vi "DefaultPsTactic.vi"(9 "Game in":refnum<class "Game.lvclass">, 10 "Robot":refnum<class "Robot.lvclass">, 11 "DefaultPsTactic in":refnum<class "DefaultPsTactic.lvclass">) -> (2 "Robot out":refnum<class "Robot.lvclass">, 3 "DefaultPsTactic out":refnum<class "DefaultPsTactic.lvclass">)   [LabVIEW 2020, in "DefaultPsTactic.lvclass"]
uses:
  DefaultPsTactic.lvclass
  C:/Users/Pedro/Dropbox/My PC (LAPTOP-06JBDO7V)/Documents/GitHub/SSL_AI/Tactic_class/Tactic.lvclass
  Robot_class/Robot.lvclass
  Game_class/Game.lvclass
  Robot_class/tactics.ctl
  Tactic_class/Tactic.lvclass/Tactic.ctl
  Game_class/Game.lvclass/Game.ctl
  Object_class/Object.lvclass/Object.ctl
  Ball_class/Ball.lvclass/Ball.ctl
  Robot_class/Robot.lvclass/Robot.ctl
  Game_class/Read BallRef.vi
  Game_class/Read Defensive ids.vi
  Object_class/Read x.vi
  Object_class/Read y.vi
  Ball_class/Read v_x.vi
  Tactic_class/Read Skillbook.vi
  Robot_class/Write tactic.vi
  Ball_class/Ball.lvclass
  C:/Users/Pedro/Dropbox/My PC (LAPTOP-06JBDO7V)/Documents/GitHub/SSL_AI/Object_class/Object.lvclass
  Skillbook_class/Skillbook.lvclass
  AttackPsSkill_class/AttackPsSkill.lvclass
  DefensePsSkill_class/DefensePsSkill.lvclass
panel:
  out "x .or. y?":bool
  out "error out":errorcluster
  in  "error in (no error)":errorcluster
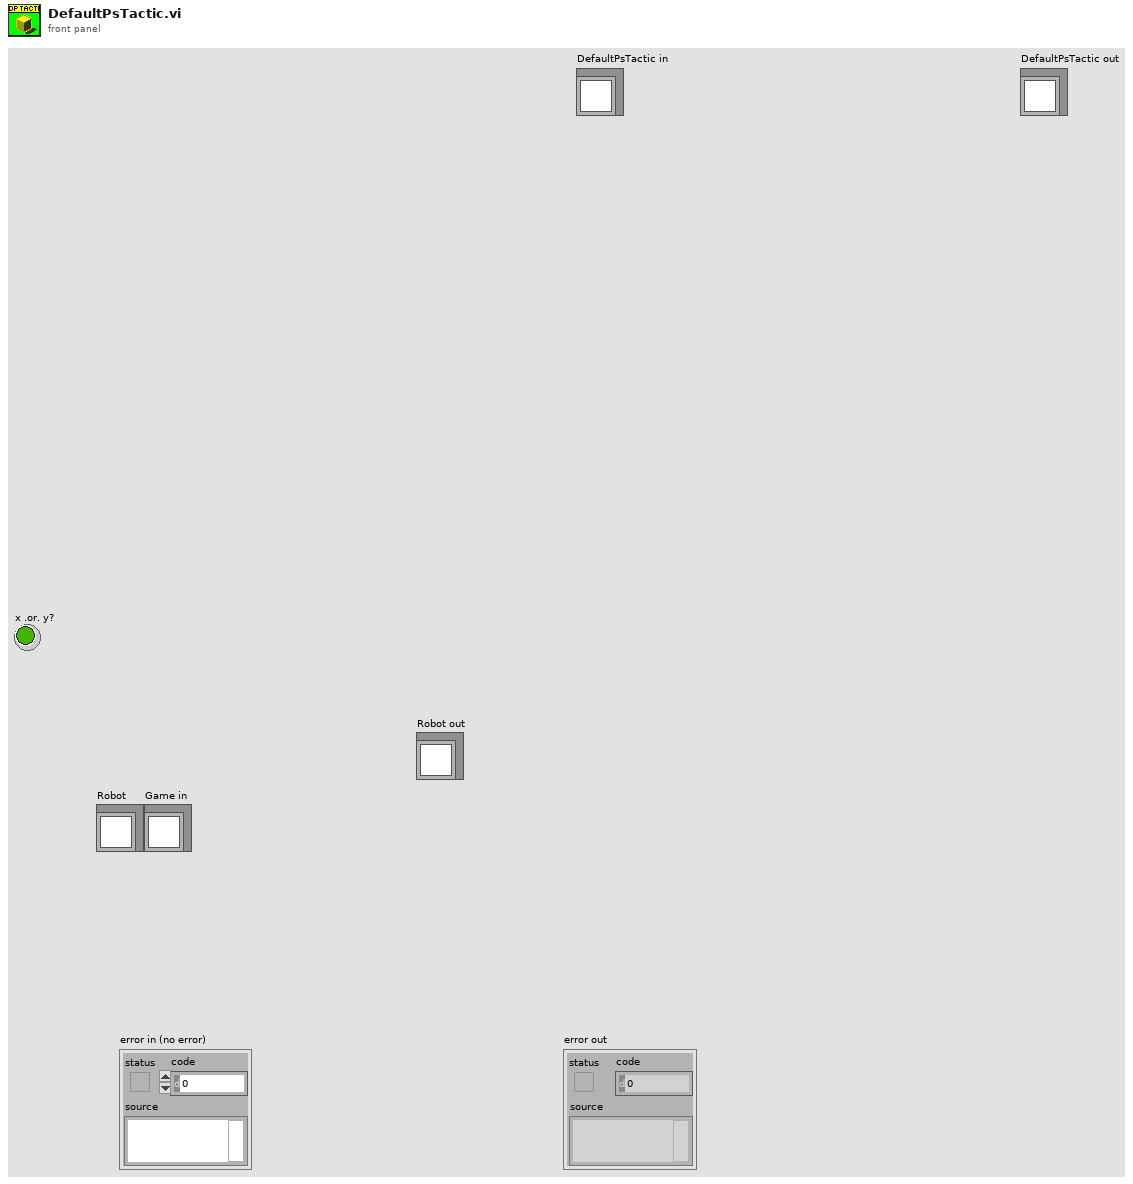
[diagram p1: front panel]
types:
  T1 = typedef "tactics.ctl" = enum16{"PenaltyAttacker", "DefaultPs", "PassObserver", "PenaltyDefense", "Test", "DefendGoal", "Marker", "FollowAttacker", "DefendArea", "Shoot", "AttackerAimGoal", "AttackerBallOutOfField", "AttackerBlock", "AttackerStop", "Duelist", "Halt", "ZigZag", "GoTo", "Timeout", "KickToPassReceiver", "PositionToReceivePass", "PassReceiver", "WaitPass"}
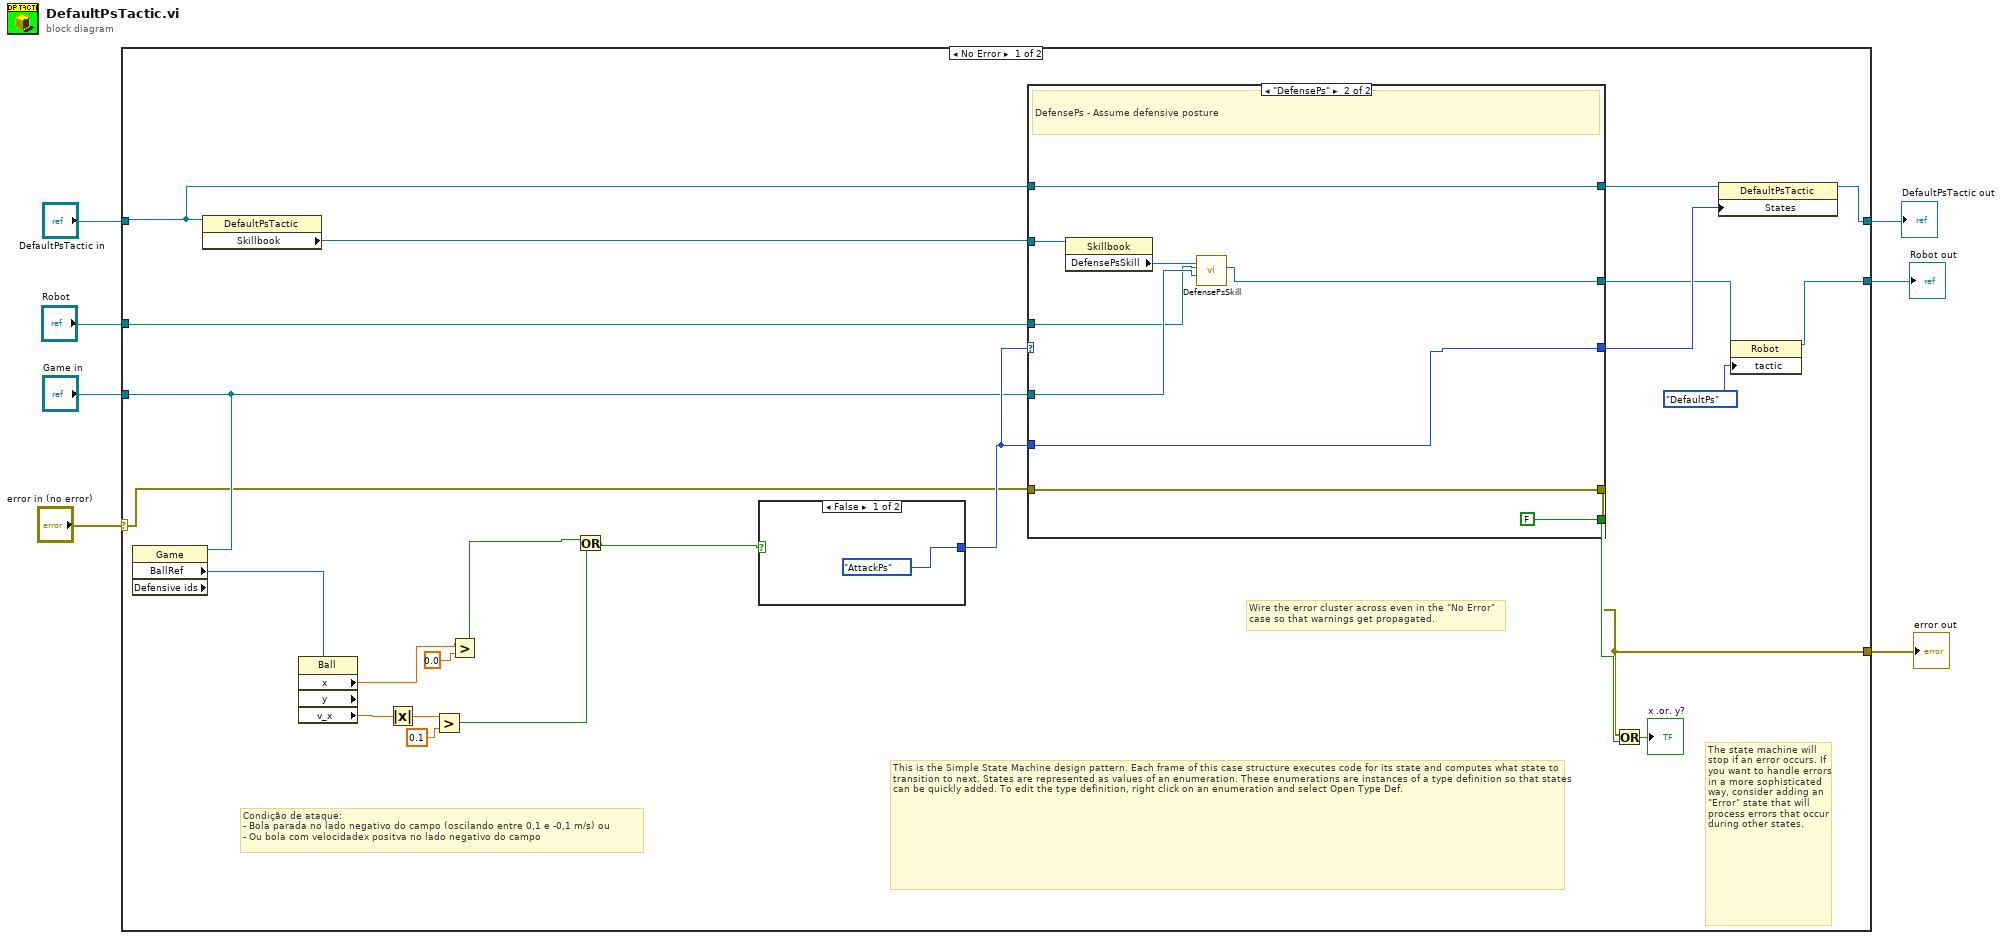
[diagram p0: block diagram]
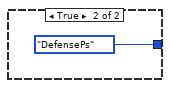
[diagram p2: hidden frame]
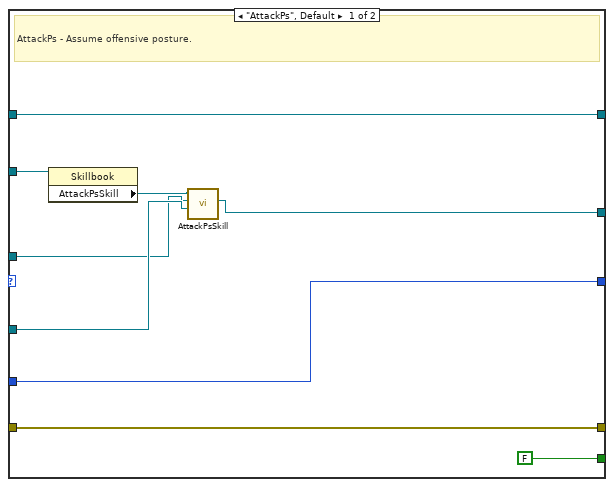
[diagram p3: hidden frame]
diagram:
  n1 = case shown="No Error" "error in (no error)" {
    selector: "error in (no error)" -> [w16 w54]
    tunnel: [w29 w54] -> w6
    tunnel: [w24 w53] -> w2
    tunnel: "DefaultPsTactic in" -> [w27 w53]
    tunnel: "Robot" -> [w28 w52]
    tunnel: [w21 w52] -> w4
    tunnel: "Game in" -> [w18 _]
    frame No Error {
      # "Condição de ataque: \n- Bola parada no lado negativo do campo (oscilando entre 0,1 e -0,1 m/s) ou\n- Ou bola com velocidadex positva no lado negativo do campo"
      # "The state machine will stop if an error occurs. If you want to handle errors in a more sophisticated way, consider adding an \"Error\" state that will process errors that occur during other states."
      # "This is the Simple State Machine design pattern. Each frame of this case structure executes code for its state and computes what state to transition to next. States are represented as values of an enumeration. These enumerations are instances of a type definition so that states can be quickly added. To edit the type definition, right click on an enumeration and select Open Type Def."
      # "Wire the error cluster across even in the \"No Error\"\ncase so that warnings get propagated."
      n2 = property class="Game" props=["BallRef", "Defensive ids"](reference=w18) -> ("BallRef"=w17:refnum<class "Ball.lvclass">)  [unwired: 1 in, 3 out]
      n3 = property class="DefaultPsTactic"(reference=w27) -> ("Skillbook"=w26:refnum<class "Skillbook.lvclass">)  [unwired: 1 in, 2 out]
      n4 = property class="Ball" props=["x", "y", "v_x"](reference=w17) -> ("x"=w13:dbl, "v_x"=w15:dbl)  [unwired: 1 in, 3 out]
      n5 = Absolute Value(x=w15) -> (abs(x)=w10:dbl)
      n6 = Greater?(x=w10, y=0.1) -> (0:w8:bool)
      n7 = Greater?(x=w13, y=0.0) -> (0:w11:bool)
      n8 = Or(x=w11, y=w8) -> (x .or. y?=w14:bool)
      n9 = case shown="False" w14 {
        tunnel: [enum16{"Exit", "AttackPs", "DefensePs"}."AttackPs" ("States") enum16{"Exit", "AttackPs", "DefensePs"}."DefensePs" ("States")] -> w19
        frame False {
        }
        frame True {
        }
      }
      n10 = case shown="\"DefensePs\"" w19 {
        tunnel: [w34 w43] -> w23
        tunnel: [FALSE ("Stop Loop?") FALSE ("Stop Loop?")] -> w31
        tunnel: w16 -> [w41 w50]
        tunnel: [w41 w50] -> w29
        tunnel: w26 -> [w40 w49]
        tunnel: w28 -> [w36 w45]
        tunnel: [w35 w44] -> w22
        tunnel: [w39 w48] -> w25
        tunnel: w27 -> [w39 w48]
        tunnel: w18 -> [w37 w46]
        tunnel: w19 -> [w34 w43]
        frame "AttackPs", Default {
          # "AttackPs - Assume offensive posture."
          n11 = property class="Skillbook"(reference=w40) -> ("AttackPsSkill"=w38:refnum<class "AttackPsSkill.lvclass">)  [unwired: 1 in, 2 out]
          n12 = call "AttackPsSkill.vi"("Game in"=w37, "Robot"=w36, "AttackPsSkill in"=w38) -> ("Robot out"=w35:refnum<class "Robot.lvclass">)  [unwired: 7 in, 1 out]
        }
        frame "DefensePs" {
          # "DefensePs - Assume defensive posture"
          n13 = property class="Skillbook"(reference=w49) -> ("DefensePsSkill"=w47:refnum<class "DefensePsSkill.lvclass">)  [unwired: 1 in, 2 out]
          n14 = call "DefensePsSkill.vi"("Game in"=w46, "Robot"=w45, "DefensePsSkill in"=w47) -> ("Robot out"=w44:refnum<class "Robot.lvclass">)  [unwired: 7 in, 1 out]
        }
      }
      n15 = Or(x=w29, y=w31) -> (x .or. y?=→"x .or. y?":bool)
      n16 = property class="DefaultPsTactic"(reference=w25, "States"=w23) -> (reference out=w24:refnum<class "DefaultPsTactic.lvclass">)  [unwired: 1 in, 1 out]
      n17 = property class="Robot"(reference=w22, "tactic"=tactics."DefaultPs") -> (reference out=w21:refnum<class "Robot.lvclass">)  [unwired: 1 in, 1 out]
    }
    frame Error {
    }
  }
  "DefaultPsTactic out" <- w2
  "error out" <- w6
  "Robot out" <- w4
